vi "Create Caster Angular Velocity Row.vi"(8 "error in (no error)":errorcluster, 11 "caster wheel in":refnum<class "NI_Robotics_Caster Wheel.lvclass">) -> (0 "error out":errorcluster, 1 "current caster angle":dbl, 2 "wheel caster angular velocity row":dbl[](array[numeric]), 3 "caster wheel out":refnum<class "NI_Robotics_Caster Wheel.lvclass">)   [LabVIEW 2017, in "NI_Robotics_Caster Wheel.lvclass"]
uses:
  <vilib>/robotics/Steering/Caster Wheel/NI_Robotics_Caster Wheel.lvclass
  c:/Program Files (x86)/National Instruments/LabVIEW 2017/vi.lib/robotics/Steering/Wheel/NI_Robotics_Wheel.lvclass
  <vilib>/robotics/Steering/Wheel/NI_Robotics_Wheel.lvclass/NI_Robotics_Wheel.ctl
  <vilib>/robotics/Steering/Caster Wheel/NI_Robotics_Caster Wheel.lvclass/NI_Robotics_Caster Wheel.ctl
  <vilib>/robotics/Steering/Wheel/NI_Robotics_Wheel.lvclass
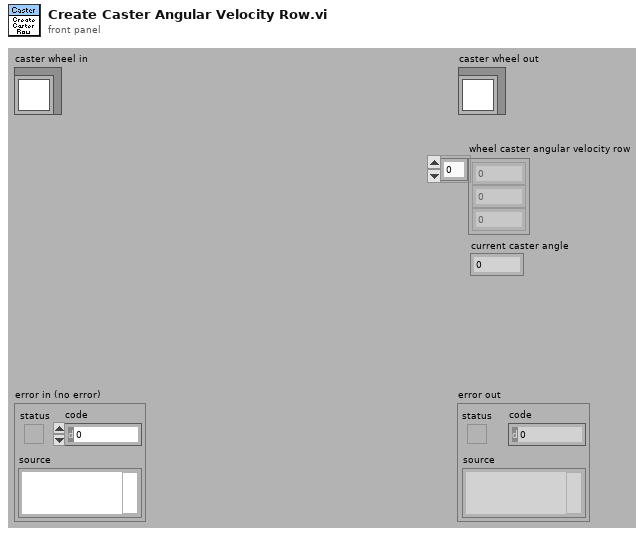
[diagram p1: front panel]
types:
  T1 = typedef "NI_Matrix.lvlib/RealMatrix.ctl" = dbl[][]
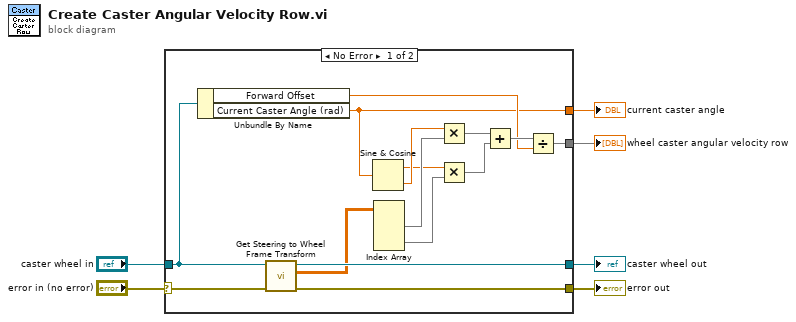
[diagram p0: block diagram]
diagram:
  n1 = case shown="No Error" "error in (no error)" {
    selector: "error in (no error)" -> [w12 w23]
    tunnel: "caster wheel in" -> [w14 w22]
    tunnel: [w11 w23] -> w4
    tunnel: [w13 w22] -> w3
    tunnel: [w15 _] -> w2
    tunnel: [w9 _] -> w1
    frame No Error {
      n2 = Unbundle By Name(w14) -> ("Forward Offset"=w16:dbl, "Current Caster Angle (rad)"=w9:dbl)
      n3 = call <vilib>:"Get Steering to Wheel Frame Transform.vi"("error in (no error)"=w12, "wheel in"=w14) -> ("error out"=w11:errorcluster, "steering to wheel frame transform"=w10:T1, "wheel out"=w13:refnum<class "NI_Robotics_Caster Wheel.lvclass">)  [unwired: 7 in]
      n4 = Sine & Cosine(0:w9) -> (1:w7:dbl, 2:w8:dbl)
      n5 = Index Array(array=w10) -> (element #1=w21:dbl[], element #2=w20:dbl[])  [unwired: 4 in]
      n6 = Multiply(x=w8, y=w21) -> (x*y=w19:dbl[])
      n7 = Multiply(x=w7, y=w20) -> (x*y=w18:dbl[])
      n8 = Add(x=w19, y=w18) -> (x+y=w17:dbl[])
      n9 = Divide(x=w17, y=w16) -> (x/y=w15:dbl[])
    }
    frame Error {
    }
  }
  "error out" <- w4
  "caster wheel out" <- w3
  "wheel caster angular velocity row" <- w2
  "current caster angle" <- w1
